vi "Normalize Connection String.vi"(10 "Destination":string, 11 "Source":string) -> (3 "Normalized Connection String":string)   [LabVIEW 2020, in "Routing and Faulting System Explorer.lvlib"]
uses:
  Routing and Faulting System Explorer.lvlib
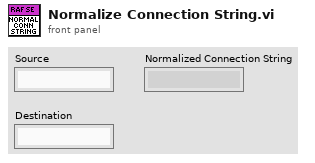
[diagram p1: front panel]
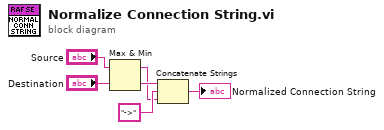
[diagram p0: block diagram]
diagram:
  n1 = Max & Min(x="Source", y="Destination") -> (max(x,y)=w2:string, min(x,y)=w4:string)
  n2 = Concatenate Strings(w4, "->" ("string"), w2) -> (→"Normalized Connection String":string)
